vi "JKI_Test.vi"() -> ()   [LabVIEW 2018]
uses:
  Typedefs/DataBuffer.ctl
  <vilib>/xnet/xnet.llb/XNET Frame CAN.ctl
  <vilib>/xnet/xnet.llb/XNET Frame Type CAN.ctl
  TEST/Typedefs/Command.ctl
  <vilib>/xnet/xnet.llb/XNET Write (Frame CAN).vi
  <vilib>/xnet/xnet.llb/XNET Read (Frame CAN).vi
panel:
  out "Event":string
  out "CAN Data":string[][](table)
  out "Response Good?":bool
  in  "SendCan":bool
  in  "OK":bool
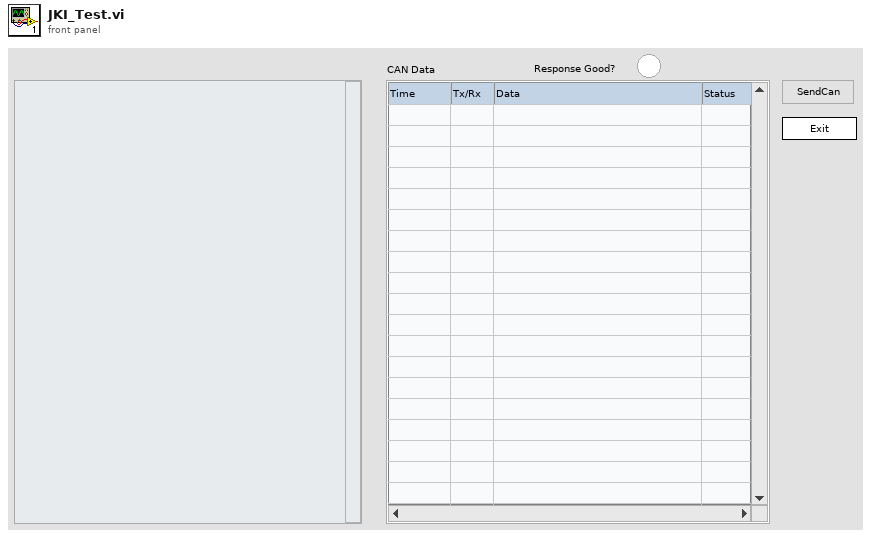
[diagram p1: front panel]
types:
  T1 = enum32{"Invalid", "Standard", "Closed", "Hidden", "Minimized", "Maximized"}
  T2 = enum32{"invalid app kind", "Development System", "Run Time System", "Student Edition", "Embedded LabVIEW", "Evaluation", "Custom"}
  T3 = typedef "DataBuffer.ctl" = cluster{"HMI":cluster{"Download Progress":refnum<vi>, "Status":refnum<vi>, "SCU Info":refnum<vi>, "PartType":refnum<vi>}, "path":path, "CAN":cluster{"Write Session in":refnum<k21>, "Read Session in":refnum<k21>, "TxRx Data":string[][], "Response Good?":bool, "spreadsheet string":string, "Rx Message":u8[], "CAN frame":T4, "HoldSession":refnum<k21>}, "error":errorcluster, "CaseControl":T6, "NewEvent":T8, "Byte Log":string[][], "Message":refnum<vi>}
  T4 = typedef "XNET Frame CAN.ctl" = cluster{"timestamp":timestamp, "payload":u8[], "identifier":u32, "type":T5, "extended?":bool, "echo?":bool}
  T5 = typedef "XNET Frame Type CAN.ctl" = u8
  T6 = typedef "CaseControl.ctl" = cluster{"histCase":cluster{"time":string, "event":T7, "pass?":bool}[], "retryCount":i32, "presentCase":T7, "nextEvent":T7}
  T7 = typedef "Command.ctl" = enum16{"Extend Session: 10 83", "Tester Present: 3E 80", "Resquest Seed: 27 01", "Send Key: 27 02", "Check FBL:  31 01 FD 02", "Control DTC: 85 82", "Comm Control: 28 83 01", "Program Session Request: 10 02", "Request Seed: 27 35", "Seed Key: 27 36", "Request Download: 34 00 44", "Transfer Data: 36 XX YY", "More Data?", "Request Transfer Exit: 37", "Check Flash Driver Validity: 01 FD 03", "More Segment?", "Write Data Fingereint: 23 F1 F0+26", "EraseFlashMemory Routine: 31 01 FD 00 44", "More segment?(each file)", "CheckAppSwAppData Validity: 31 01 FD 04 44", "CheckAppSwAppData Dependency: 31 01 fd 01", "ECU Reset: 11 81", "System: Init", "System: Idle", "System: Error", "System: Wait", "System: Delay", "System: CAN Send 1", "System: CAN Send 2", "System: CAN Read", "System: Exit"}
  T8 = typedef "NewEvent.ctl" = cluster{"Delay_ms":i32, "Case":T7, "Payload":u8[], "Identifier":u32}
  T9 = cluster{"Core":cluster{"Current VI Reference":refnum<vi>, "Close Panel on Exit?":bool}, "Your Boolean data":bool, "Event":string, "Hist Event":string, "DataBuffer":T3, "Delay_ms":u32}
  T10 = cluster{"Current VI Reference":refnum<vi>, "Close Panel on Exit?":bool}
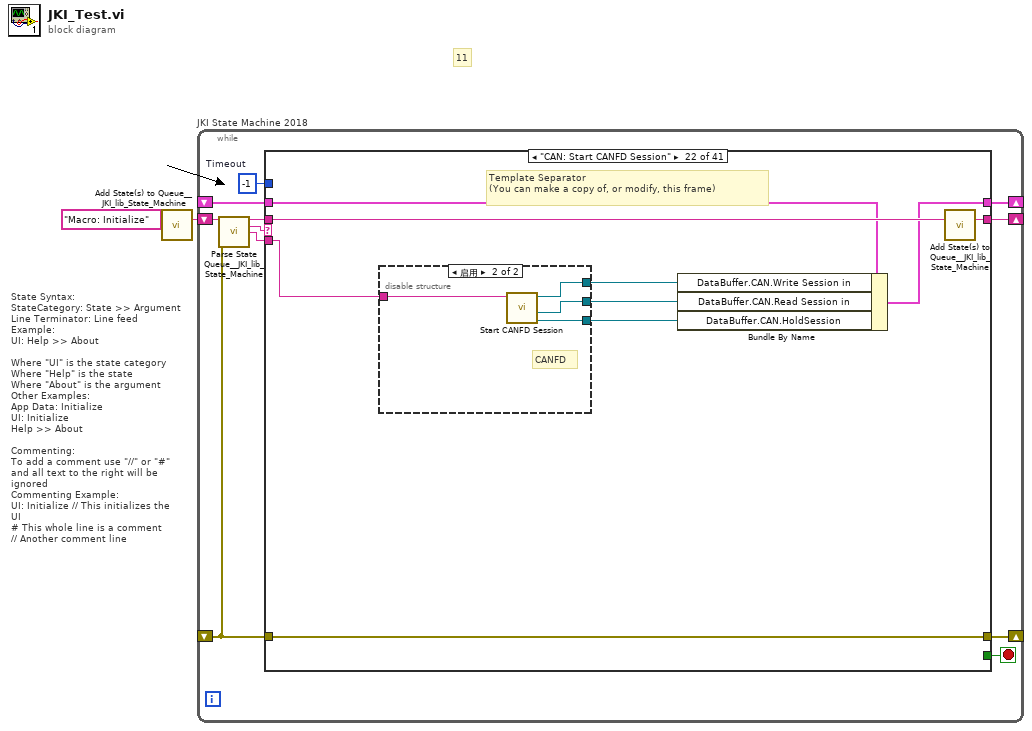
[diagram p0: block diagram]
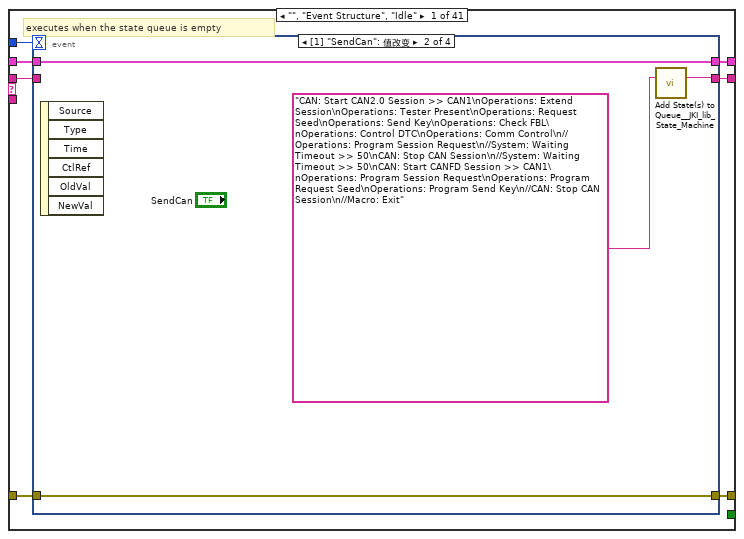
[diagram p2: hidden frame]
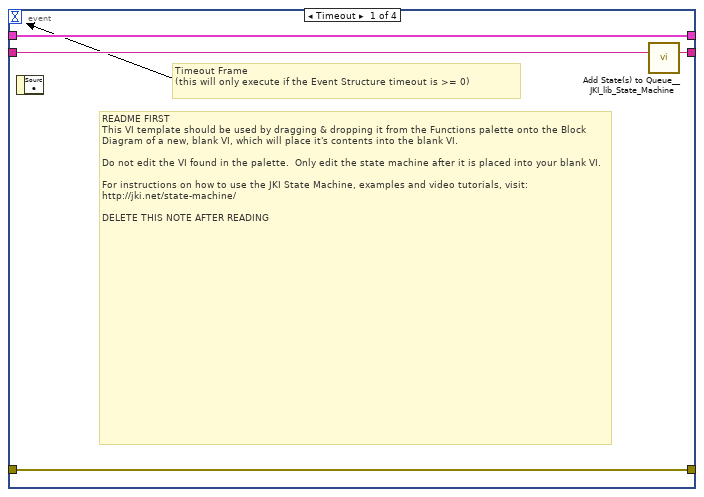
[diagram p3: hidden frame]
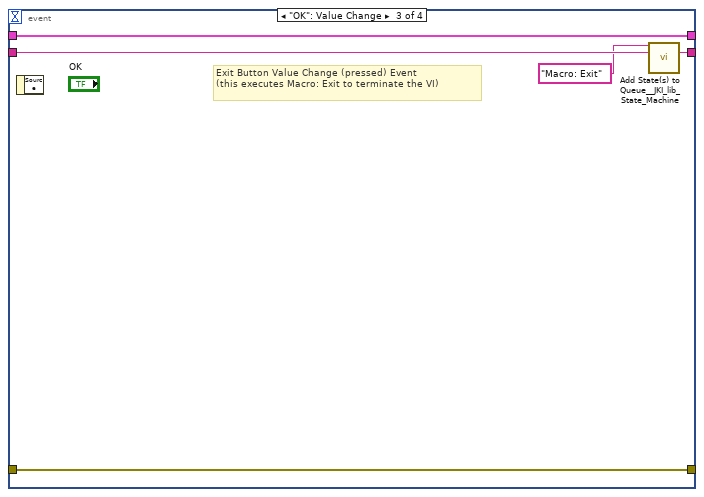
[diagram p4: hidden frame]
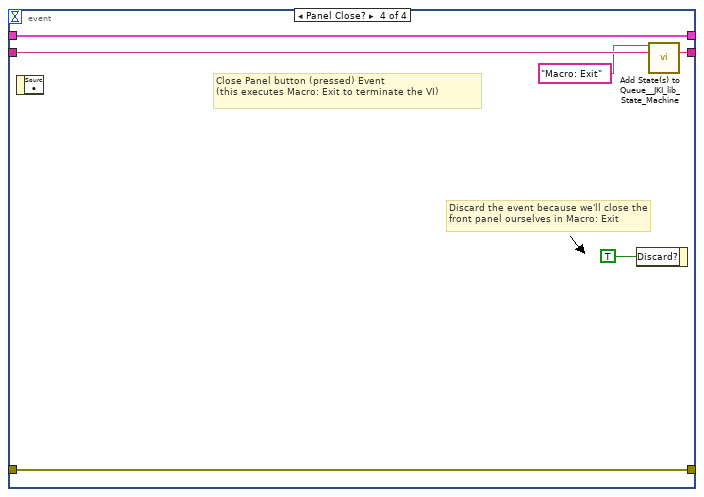
[diagram p5: hidden frame]
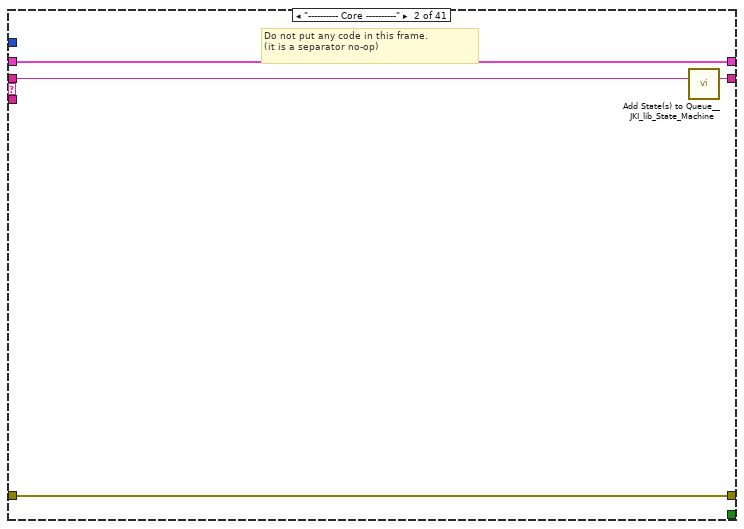
[diagram p6: hidden frame]
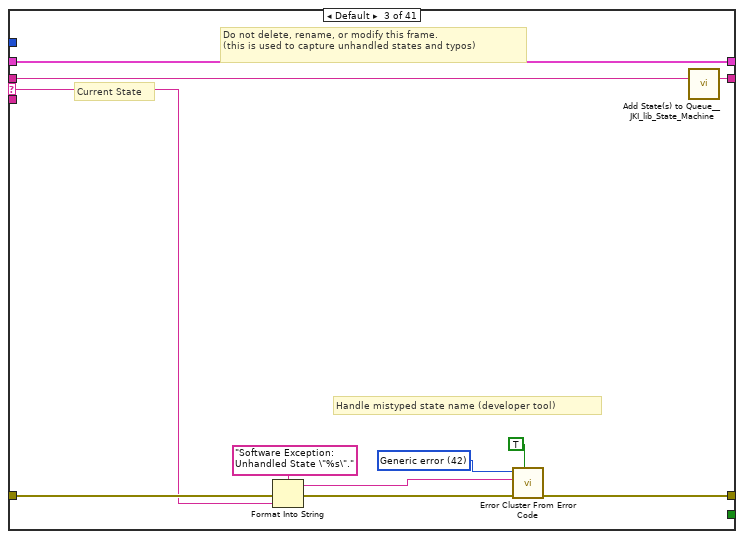
[diagram p7: hidden frame]
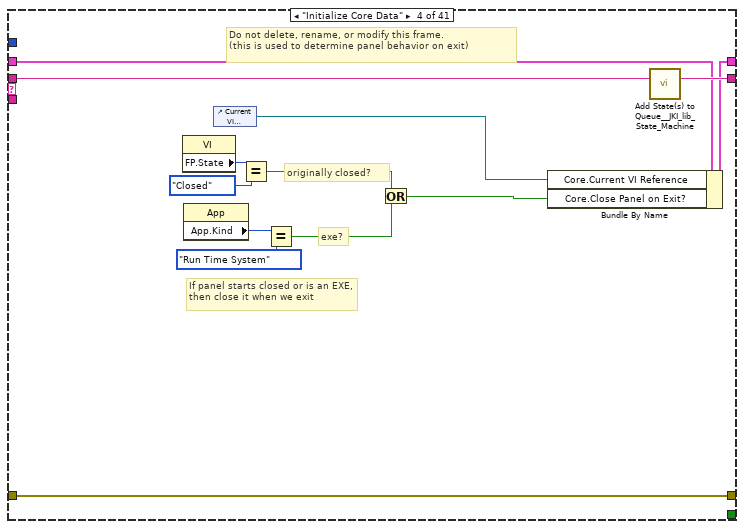
[diagram p8: hidden frame]
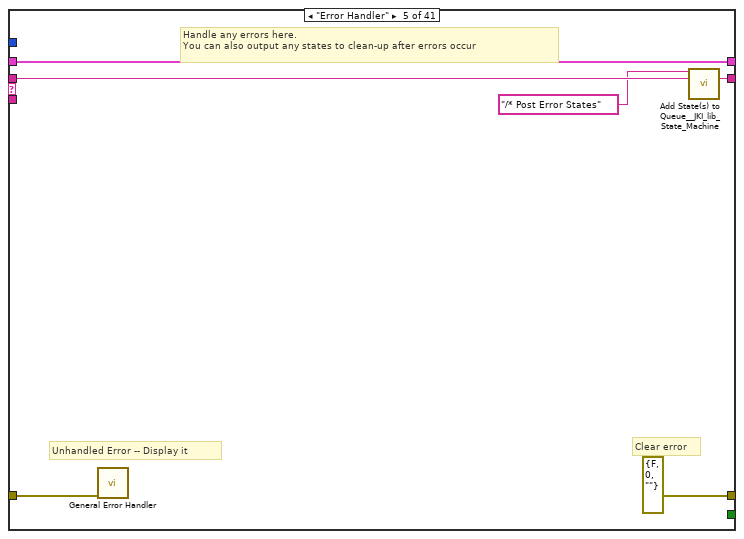
[diagram p9: hidden frame]
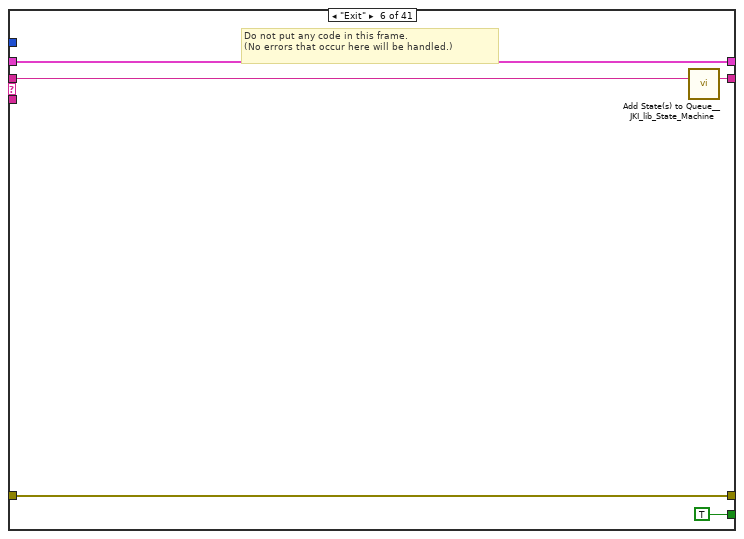
[diagram p10: hidden frame]
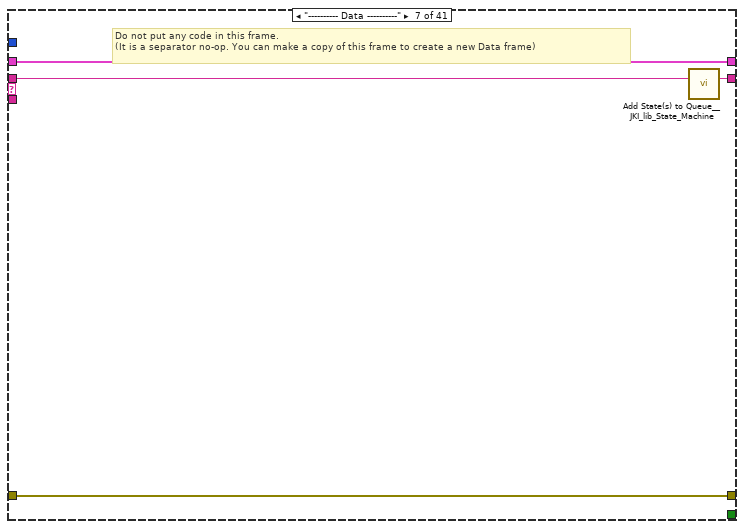
[diagram p11: hidden frame]
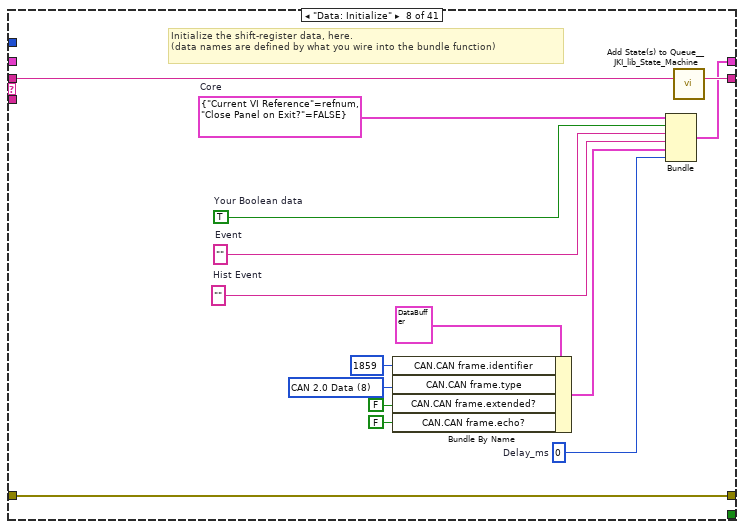
[diagram p12: hidden frame]
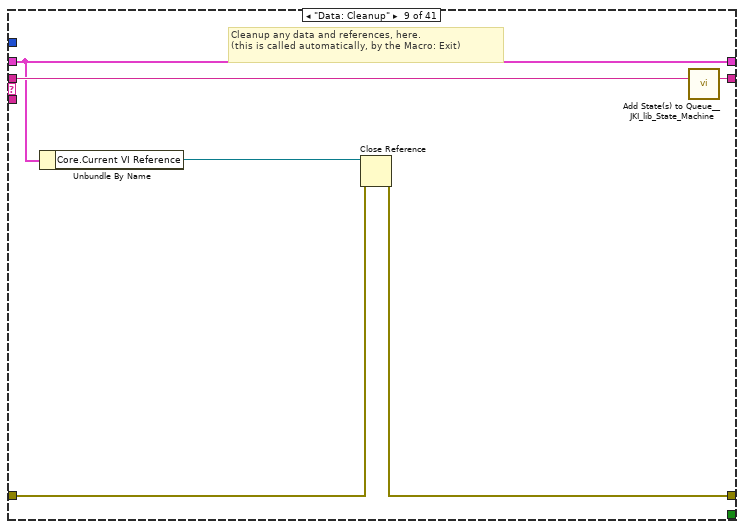
[diagram p13: hidden frame]
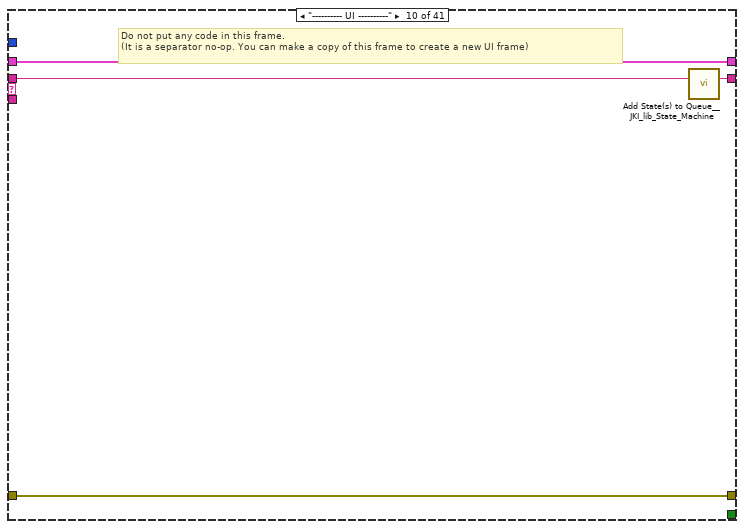
[diagram p14: hidden frame]
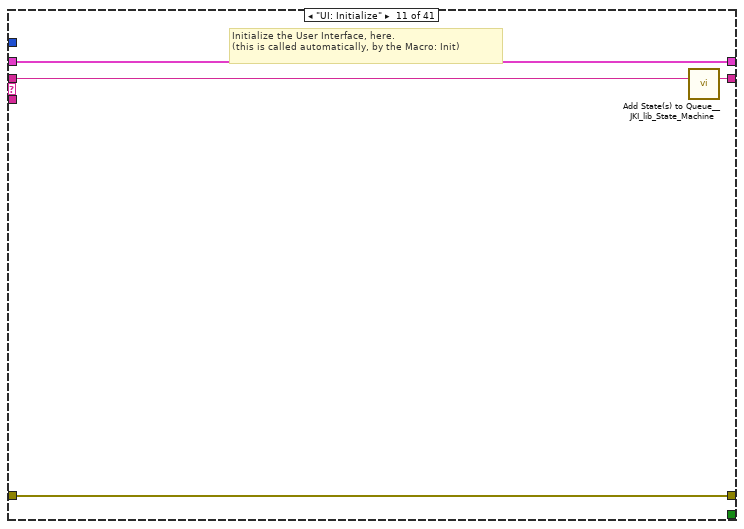
[diagram p15: hidden frame]
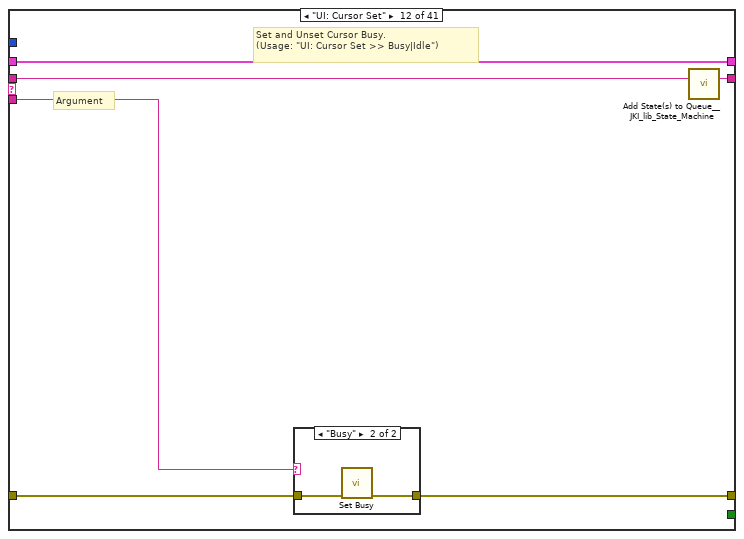
[diagram p16: hidden frame]
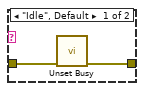
[diagram p17: hidden frame]
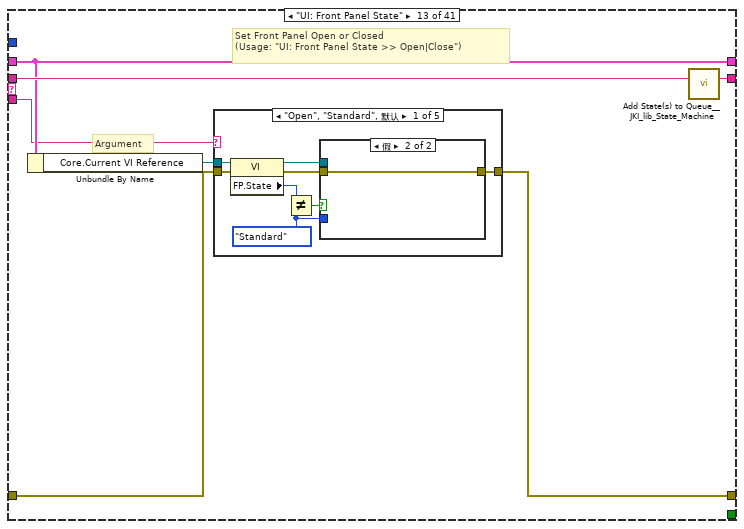
[diagram p18: hidden frame]
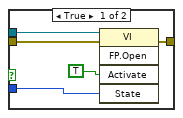
[diagram p19: hidden frame]
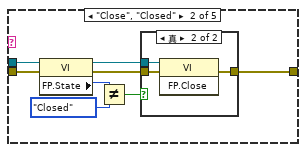
[diagram p20: hidden frame]
diagram:
  # "11"
  # "State Syntax:\nStateCategory: State >> Argument\nLine Terminator: Line feed\nExample:\nUI: Help >> About\n\nWhere \"UI\" is the state category\nWhere \"Help\" is the state\nWhere \"About\" is the argument\nOther Examples:\nApp Data: Initialize\nUI: Initialize\nHelp >> About\n\nCommenting:\nTo add a comment use \"//\" or \"#\" and all text to the right will be ignored\nCommenting Example:\nUI: Initialize // This initializes the UI\n# This whole line is a comment\n// Another comment line"
  n1 = call <vilib>:"Add State(s) to Queue__JKI_lib_State_Machine.vi"("State(s) in (\"\")"="Macro: Initialize") -> ("States Out"=w2:string)  [unwired: 14 in]
  n2 = while "JKI State Machine 2018" {
    shift-right: [w6] -> _
    shift-left: _ -> [w5]
    shift-right: [w9] -> _
    shift-left: _ -> [w3]
    shift-right: [w8] -> _
    shift-left: w2 -> [w10]
    stop <- w7 stop-if-true
    w4 = -1  # Timeout
    n3 = call <vilib>:"Parse State Queue__JKI_lib_State_Machine.vi"("State Queue"=w10, "Error In (no error)"=w3) -> ("Remaining States"=w12:string, "Current State"=w13:string, "Arguments"=w11:string)  [unwired: 11 in]
    n4 = case shown="\"CAN: Start CANFD Session\"" w13 {
      selector: w13 -> [_ _ w44 _ _ _ _ _ _ _ _ _ _ _ _ _ _ _ _ _ _ _ _ _ _ _ _ _ _ _ _ w363 w383 w404 w424 w448 w468 w491 w511 w532 w553]
      tunnel: w12 -> [w20 w43 w48 w67 w73 w78 w82 w97 w103 w107 w111 w117 w128 w197 w202 w212 w216 w236 w250 w254 w263 w279 w301 w319 w333 w339 w343 w347 w351 w355 w359 w380 w401 w421 w445 w465 w486 w506 w527 w549 w574]
      tunnel: w11 -> [_ _ _ _ _ _ _ _ _ _ _ w112 w122 _ _ _ _ _ w240 _ w257 w273 w295 _ _ _ _ _ _ _ _ w361 w382 w403 w423 w447 w467 w490 w510 w531 w552]
      tunnel: w5 -> [w18 w40 w46 w60 w70 w76 w79 _ w98 w104 w109 w115 w124 w194 w199 w209 w213 w233 w247 w251 w261 w277 w298 w316 w331 w336 w340 w344 w348 w352 w356 w372 w393 w413 w437 w457 w478 w498 w519 w541 w566]
      tunnel: [w17 w41 w50 w64 errorcluster {"status"=FALSE, "code"=0, "source"=""} ("error out") w75 w80 w94 w99 w105 w108 w113 w125 w195 w200 w210 w214 w234 w248 w252 w255 w271 w299 w317 w327 w337 w341 w345 w349 w353 w357 w378 w399 w419 w443 w463 w484 w504 w525 w547 w572] -> w9
      tunnel: w3 -> [w16 w41 w49 w64 w69 w75 w80 w94 w100 w105 w108 w114 w126 w195 w200 w210 w214 _ w248 w252 w255 w271 w299 w317 w327 w337 w341 w345 w349 w353 w357 w378 w399 w419 w443 w463 w484 w504 w525 w547 w572]
      tunnel: [w19 w42 w47 w66 w72 w77 w81 w96 w102 w106 w110 w116 w127 w196 w201 w211 w215 w235 w249 w253 w262 w278 w300 w318 w332 w338 w342 w346 w350 w354 w358 w379 w400 w420 w444 w464 w485 w505 w526 w548 w573] -> w8
      tunnel: [_ _ _ _ _ TRUE _ _ _ _ _ _ _ _ _ _ _ _ _ _ _ _ _ _ _ _ _ _ _ _ _ _ _ _ _ _ _ _ _ _ _] -> w7
      tunnel: [w15 w40 w46 w65 w70 w76 w79 w95 w98 w104 w109 w115 w124 w194 w199 w209 w213 w232 w247 w251 w260 w276 w297 w316 w331 w336 w340 w344 w348 w352 w356 w371 w392 w412 w436 w456 w477 w497 w518 w540 w565] -> w6
      tunnel: w4 -> [w14 _ _ _ _ _ _ _ _ _ _ _ _ _ _ _ _ _ _ _ _ _ _ _ _ _ _ _ _ _ _ _ _ _ _ _ _ _ _ _ _]
      frame "", "Event Structure", "Idle" {
        # "executes when the state queue is empty"
        n5 = event shown="[1] \"SendCan\": 值改变" {
          selector: _ -> [_ _ _ _]
          dyn-events: _ -> [_ _ _ _]
          timeout: w14 -> [_ _ _ _]
          tunnel: w20 -> [w24 _ w33 w39]
          tunnel: [w23 w27 w32 w38] -> w19
          tunnel: w18 -> [w21 w28 w30 w36]
          tunnel: [w22 w26 w31 w37] -> w17
          tunnel: w16 -> [w22 w26 w31 w37]
          tunnel: [w21 w28 w30 w36] -> w15
          event Timeout {
            # "README FIRST\nThis VI template should be used by dragging & dropping it from the Functions palette onto the Block Diagram of a new, blank VI, which will place it's contents into the blank VI.\n\nDo not edit the VI found in the palette.  Only edit the state machine after it is placed into your blank VI.\n\nFor instructions on how to use the JKI State Machine, examples and video tutorials, visit:\nhttp://jki.net/state-machine/\n\nDELETE THIS NOTE AFTER READING"
            # "Timeout Frame\n(this will only execute if the Event Structure timeout is >= 0)"
            n6 = event-data() -> ()  [unwired: 1 in, 1 out]
            n7 = call <vilib>:"Add State(s) to Queue__JKI_lib_State_Machine.vi"("State(s) in (\"\")"=w24) -> ("States Out"=w23:string)  [unwired: 14 in]
          }
          event "SendCan": Value Change {
            n8 = event-data() -> ()  [unwired: 1 in, 6 out]
            n9 = call <vilib>:"Add State(s) to Queue__JKI_lib_State_Machine.vi"("State(s) in (\"\")"="CAN: Start CAN2.0 Session >> CAN1\nOperations: Extend Session\nOperations: Tester Present\nOperations: Request Seed\nOperations: Send Key\nOperations: Check FBL\nOperations: Control DTC\nOperations: Comm Control\n//Operations: Program Session Request\n//System: Waiting Timeout >> 50\nCAN: Stop CAN Session\n//System: Waiting Timeout >> 50\nCAN: Start CANFD Session >> CAN1\nOperations: Program Session Request\nOperations: Program Request Seed\nOperations: Program Send Key\n//CAN: Stop CAN Session\n//Macro: Exit") -> ("States Out"=w27:string)  [unwired: 14 in]
          }
          event "OK": Value Change {
            # "Exit Button Value Change (pressed) Event\n(this executes Macro: Exit to terminate the VI)"
            n10 = event-data() -> ()  [unwired: 1 in, 1 out]
            n11 = call <vilib>:"Add State(s) to Queue__JKI_lib_State_Machine.vi"("State(s) in Front (\"\")"="Macro: Exit", "State(s) in (\"\")"=w33) -> ("States Out"=w32:string)  [unwired: 13 in]
          }
          event Panel Close? {
            # "Discard the event because we'll close the front panel ourselves in Macro: Exit"
            # "Close Panel button (pressed) Event\n(this executes Macro: Exit to terminate the VI)"
            n12 = event-data() -> ()  [unwired: 1 in, 1 out]
            n13 = event-data("Discard?"=TRUE) -> ()  [unwired: 1 in, 1 out]
            n14 = call <vilib>:"Add State(s) to Queue__JKI_lib_State_Machine.vi"("State(s) in Front (\"\")"="Macro: Exit", "State(s) in (\"\")"=w39) -> ("States Out"=w38:string)  [unwired: 13 in]
          }
        }
      }
      frame "---------- Core ----------" {
        # "Do not put any code in this frame.\n(it is a separator no-op)"
        n15 = call <vilib>:"Add State(s) to Queue__JKI_lib_State_Machine.vi"("State(s) in (\"\")"=w43) -> ("States Out"=w42:string)  [unwired: 14 in]
      }
      frame Default {
        w53 = 42 items=["No error", "Argument error", "Memory is full", "Out of zone", "End of file", "File already open", "Generic file I/O error", "File not found", "File permission error", "Disk is full", "Duplicate path", "Too many files open", "System feature not enabled", "Resource file not found", "Cannot add resource", "Resource not found", "Image not found", "Image memory error", "Pen does not exist", "Config type invalid", "Config token not found", "Config parse error", "Config memory error", "Bad external code format", "Bad external code offset", "External code not present", "Null window", "Destroy window error", "Null menu", "Print aborted", "Bad print record", "Print driver error", "Windows error during printing", "Memory error during printing", "Print dialog error", "Generic print error", "Invalid device refnum", "Device not found", "Device parameter error", "Device unit error", "Cannot open device", "Device call aborted", "Generic error", "Cancelled by user", "Object ID too low", "Object ID too high", "Object not in heap", "Unknown heap", "Unknown object (invalid DefProc)", "Unknown object (DefProc not in table)", "Message out of range", "Invalid (null) method", "Unknown message", "Manager call not supported", "Bad address", "Network operation in progress", "Network operation timed out", "Connection is busy", "Network attribute not supported", "Network error", "Address in use", "System out of memory", "Connection aborted", "Connection refused", "Not connected", "Already connected", "Connection closed", "Initialization error (interapplication manager)", "Bad occurrence", "Wait on unbound occurrence handler", "Occurrence queue overflow", "Datalog type conflict", "Unused", "Unrecognized type (interapplication manager)", "Memory corrupt", "Failed to make temporary DLL", "Old CIN version", "Drag socket not found", "Failed to load drop-object", "Failed to register OLE object", "Failed to release OLE object", "Format specifier type mismatch", "Unknown format specifier", "Too few format specifiers", "Too many format specifiers", "Scan failed", "Newer CIN version", "Error converting to variant", "Runtime menu error", "Password tampered", "Variant attribute not found", "Incompatible variant data type", "Event data is not available", "Event Store is not present", "Occurrence is not found", "Event Queue is not created", "Event info is not available", "Refnum passed is NULL", "Error retrieving Class GUID", "Error retrieving CoClass GUID", "Error retrieving TypeLib GUID.", "Bad built application magic bytes.", "Specific driver is different from the specific driver associated with the Logical Name.", "There is no session opened to the class driver.", "Max Error", "MAX - Error with config objects", "MAX - Error loading configuration", "MAX - Group not supported"]
        # "Current State"
        # "Do not delete, rename, or modify this frame.\n(this is used to capture unhandled states and typos)"
        # "Handle mistyped state name (developer tool)"
        n16 = Format Into String(format string="Software Exception: Unhandled State \"%s\"." ("message"), error in=w49, w44) -> (resulting string=w52:string, error out=w51:errorcluster)  [unwired: 1 in]
        n17 = call <vilib>:"Error Cluster From Error Code.vi"("show call chain? (False)"=TRUE, "error in (no error)"=w51, "error message (\"\")"=w52, "error code (0)"=w53) -> ("error out"=w50:errorcluster)  [unwired: 5 in]
        n18 = call <vilib>:"Add State(s) to Queue__JKI_lib_State_Machine.vi"("State(s) in (\"\")"=w48) -> ("States Out"=w47:string)  [unwired: 14 in]
      }
      frame "Initialize Core Data" {
        # "Do not delete, rename, or modify this frame.\n(this is used to determine panel behavior on exit)"
        # "originally closed?"
        # "exe?"
        # "If panel starts closed or is an EXE, then close it when we exit"
        n19 = property class="VI"() -> ("FP.State"=w57:T1)  [unwired: 2 in, 2 out]
        n20 = property class="App"() -> ("App.Kind"=w63:T2)  [unwired: 2 in, 2 out]
        n21 = control-ref of="Current VI Reference"() -> (w58:refnum<vi>)
        n22 = Equal?(x=w57, y=T1."Closed" ("Front Panel Window:State")) -> (x = y?=w55:bool)
        n23 = Equal?(x=w63, y=T2."Run Time System" ("Application:Kind")) -> (x = y?=w61:bool)
        n24 = Or(x=w55, y=w61) -> (x .or. y?=w59:bool)
        n25 = Bundle By Name(cluster=w60, "Core.Current VI Reference"=w58, "Core.Close Panel on Exit?"=w59) -> (w65:T9)
        n26 = call <vilib>:"Add State(s) to Queue__JKI_lib_State_Machine.vi"("State(s) in (\"\")"=w67) -> ("States Out"=w66:string)  [unwired: 14 in]
      }
      frame "Error Handler" {
        # "Unhandled Error -- Display it"
        # "Handle any errors here.\nYou can also output any states to clean-up after errors occur"
        # "Clear error"
        n27 = call <vilib>:"General Error Handler.vi"("error in (no error)"=w69) -> ()  [unwired: 10 in, 5 out]
        n28 = call <vilib>:"Add State(s) to Queue__JKI_lib_State_Machine.vi"("State(s) in Front (\"\")"="/* Post Error States", "State(s) in (\"\")"=w73) -> ("States Out"=w72:string)  [unwired: 13 in]
      }
      frame "Exit" {
        # "Do not put any code in this frame.\n(No errors that occur here will be handled.)"
        n29 = call <vilib>:"Add State(s) to Queue__JKI_lib_State_Machine.vi"("State(s) in (\"\")"=w78) -> ("States Out"=w77:string)  [unwired: 14 in]
      }
      frame "---------- Data ----------" {
        # "Do not put any code in this frame.\n(It is a separator no-op. You can make a copy of this frame to create a new Data frame)"
        n30 = call <vilib>:"Add State(s) to Queue__JKI_lib_State_Machine.vi"("State(s) in (\"\")"=w82) -> ("States Out"=w81:string)  [unwired: 14 in]
      }
      frame "Data: Initialize" {
        w83 = u32 0  # Delay_ms
        w84 = ""  # Hist Event
        w87 = T5 8 items=["CAN Data"=0, "CAN Remote"=1, "CAN Bus Error"=2, "CAN 2.0 Data"=8, "CAN FD Data"=16, "CAN FD+BRS Data"=24, "J1939 Data"=192, "Delay"=224, "Log Trigger"=225, "Start Trigger"=226] ("CAN.CAN frame.type")
        w91 = T10 {"Current VI Reference"=refnum, "Close Panel on Exit?"=FALSE}  # Core
        w93 = TRUE  # Your Boolean data
        w92 = ""  # Event
        # "Initialize the shift-register data, here.\n(data names are defined by what you wire into the bundle function)"
        n31 = Bundle By Name(cluster=T3 {"HMI"={"Download Progress"=refnum, "Status"=refnum, "SCU Info"=refnum, "PartType"=refnum}, "path"=path "", "CAN"={"Write Session in"="", "Read Session in"="", "TxRx Data"=[], "Response Good?"=FALSE, "spreadsheet string"="", "Rx Message"=[], "CAN frame"={"timestamp"=timestamp(0 s since 1904-01-01), "payload"=[2, 39, 3, 85, 85, 85, 85, 85], "identifier"=402391172, "type"=16, "extended?"=TRUE, "echo?"=FALSE}, "HoldSession"=""}, "error"={"status"=FALSE, "code"=0, "source"=""}, "CaseControl"={"histCase"=[], "retryCount"=0, "presentCase"=enum."Extend Session: 10 83", "nextEvent"=enum."Extend Session: 10 83"}, "NewEvent"={"Delay_ms"=0, "Case"=enum."Extend Session: 10 83", "Payload"=[], "Identifier"=0}, "Byte Log"=[], "Message"=refnum} ("DataBuffer"), "CAN.CAN frame.identifier"=u32 1859, "CAN.CAN frame.type"=w87, "CAN.CAN frame.extended?"=FALSE, "CAN.CAN frame.echo?"=FALSE) -> (w89:T3)
        n32 = Bundle("Core"=w91, "Your Boolean data"=w93, "Event"=w92, "Hist Event"=w84, "DataBuffer"=w89, "Delay_ms"=w83) -> (w95:T9)  [unwired: 1 in]
        n33 = call <vilib>:"Add State(s) to Queue__JKI_lib_State_Machine.vi"("State(s) in (\"\")"=w97) -> ("States Out"=w96:string)  [unwired: 14 in]
      }
      frame "Data: Cleanup" {
        # "Cleanup any data and references, here.\n(this is called automatically, by the Macro: Exit)"
        n34 = Unbundle By Name(w98) -> ("Core.Current VI Reference"=w101:refnum<vi>)
        n35 = Close Reference(reference=w101, error in (no error)=w100) -> (error out=w99:errorcluster)
        n36 = call <vilib>:"Add State(s) to Queue__JKI_lib_State_Machine.vi"("State(s) in (\"\")"=w103) -> ("States Out"=w102:string)  [unwired: 14 in]
      }
      frame "---------- UI ----------" {
        # "Do not put any code in this frame.\n(It is a separator no-op. You can make a copy of this frame to create a new UI frame)"
        n37 = call <vilib>:"Add State(s) to Queue__JKI_lib_State_Machine.vi"("State(s) in (\"\")"=w107) -> ("States Out"=w106:string)  [unwired: 14 in]
      }
      frame "UI: Initialize" {
        # "Initialize the User Interface, here.\n(this is called automatically, by the Macro: Init)"
        n38 = call <vilib>:"Add State(s) to Queue__JKI_lib_State_Machine.vi"("State(s) in (\"\")"=w111) -> ("States Out"=w110:string)  [unwired: 14 in]
      }
      frame "UI: Cursor Set" {
        # "Argument"
        # "Set and Unset Cursor Busy.\n(Usage: \"UI: Cursor Set >> Busy|Idle\")"
        n39 = case shown="\"Busy\"" w112 {
          tunnel: w114 -> [w119 w121]
          tunnel: [w118 w120] -> w113
          frame "Idle", Default {
            n40 = call <vilib>:"Unset Busy.vi"("error in (no error)"=w119) -> ("error out"=w118:errorcluster)  [unwired: 10 in]
          }
          frame "Busy" {
            n41 = call <vilib>:"Set Busy.vi"("error in (no error)"=w121) -> ("error out"=w120:errorcluster)  [unwired: 9 in, 1 out]
          }
        }
        n42 = call <vilib>:"Add State(s) to Queue__JKI_lib_State_Machine.vi"("State(s) in (\"\")"=w117) -> ("States Out"=w116:string)  [unwired: 14 in]
      }
      frame "UI: Front Panel State" {
        # "Argument"
        # "Set Front Panel Open or Closed\n(Usage: \"UI: Front Panel State >> Open|Close\")"
        n43 = Unbundle By Name(w124) -> ("Core.Current VI Reference"=w123:refnum<vi>)
        n44 = case shown="\"Open\", \"Standard\", 默认" w122 {
          tunnel: w126 -> [w134 w149 w160 w173 w186]
          tunnel: [w136 w150 w162 w175 w188] -> w125
          tunnel: w123 -> [w135 w147 w161 w174 w187]
          frame "Open", "Standard", Default {
            w129 = T1."Standard" ("State")
            n45 = property class="VI"(reference=w135, error in=w134) -> (reference out=w132:refnum<vi>, error out=w133:errorcluster, "FP.State"=w131:T1)
            n46 = Not Equal?(x=w131, y=w129) -> (x != y?=w130:bool)
            n47 = case shown="假" w130 {
              tunnel: [w140 w142] -> w136
              tunnel: w133 -> [w139 w142]
              tunnel: w132 -> [w138 _]
              tunnel: w129 -> [w137 _]
              frame True {
                n48 = invoke class="VI" method="FP.Open"(reference=w138, error in=w139, "Activate"=TRUE, "State"=w137) -> (error out=w140:errorcluster)  [unwired: 1 in, 4 out]
              }
              frame False {
              }
            }
          }
          frame "Close", "Closed" {
            n49 = property class="VI"(reference=w147, error in=w149) -> (reference out=w146:refnum<vi>, error out=w148:errorcluster, "FP.State"=w144:T1)
            n50 = Not Equal?(x=w144, y=T1."Closed" ("Front Panel Window:State")) -> (x != y?=w143:bool)
            n51 = case shown="真" w143 {
              tunnel: [w151 w154] -> w150
              tunnel: w148 -> [w151 w153]
              tunnel: w146 -> [_ w152]
              frame False {
              }
              frame True {
                n52 = invoke class="VI" method="FP.Close"(reference=w152, error in=w153) -> (error out=w154:errorcluster)  [unwired: 1 in, 2 out]
              }
            }
          }
          frame "Hidden", "Hide" {
            w155 = T1."Hidden" ("State")
            n53 = property class="VI"(reference=w161, error in=w160) -> (reference out=w158:refnum<vi>, error out=w159:errorcluster, "FP.State"=w157:T1)
            n54 = Not Equal?(x=w157, y=w155) -> (x != y?=w156:bool)
            n55 = case shown="假" w156 {
              tunnel: [w166 w167] -> w162
              tunnel: w159 -> [w165 w167]
              tunnel: w158 -> [w164 _]
              tunnel: w155 -> [w163 _]
              frame True {
                n56 = invoke class="VI" method="FP.Open"(reference=w164, error in=w165, "State"=w163) -> (error out=w166:errorcluster)  [unwired: 2 in, 4 out]
              }
              frame False {
              }
            }
          }
          frame "Minimize", "Minimized" {
            w168 = T1."Minimized" ("State")
            n57 = property class="VI"(reference=w174, error in=w173) -> (reference out=w171:refnum<vi>, error out=w172:errorcluster, "FP.State"=w170:T1)
            n58 = Not Equal?(x=w170, y=w168) -> (x != y?=w169:bool)
            n59 = case shown="真" w169 {
              tunnel: [w179 w180] -> w175
              tunnel: w172 -> [w178 w180]
              tunnel: w171 -> [w177 _]
              tunnel: w168 -> [w176 _]
              frame True {
                n60 = invoke class="VI" method="FP.Open"(reference=w177, error in=w178, "State"=w176) -> (error out=w179:errorcluster)  [unwired: 2 in, 4 out]
              }
              frame False {
              }
            }
          }
          frame "Maximize", "Maximized" {
            w181 = T1."Maximized" ("State")
            n61 = property class="VI"(reference=w187, error in=w186) -> (reference out=w184:refnum<vi>, error out=w185:errorcluster, "FP.State"=w183:T1)
            n62 = Not Equal?(x=w183, y=w181) -> (x != y?=w182:bool)
            n63 = case shown="真" w182 {
              tunnel: [w192 w193] -> w188
              tunnel: w185 -> [w191 w193]
              tunnel: w184 -> [w190 _]
              tunnel: w181 -> [w189 _]
              frame True {
                n64 = invoke class="VI" method="FP.Open"(reference=w190, error in=w191, "State"=w189) -> (error out=w192:errorcluster)  [unwired: 2 in, 4 out]
              }
              frame False {
              }
            }
          }
        }
        n65 = call <vilib>:"Add State(s) to Queue__JKI_lib_State_Machine.vi"("State(s) in (\"\")"=w128) -> ("States Out"=w127:string)  [unwired: 14 in]
      }
      frame "---------- Macro ----------" {
        # "Do not put any code in this frame.\n(It is a separator no-op. You can make a copy of this frame to create a new Macro frame)"
        n66 = call <vilib>:"Add State(s) to Queue__JKI_lib_State_Machine.vi"("State(s) in (\"\")"=w197) -> ("States Out"=w196:string)  [unwired: 14 in]
      }
      frame "Macro: Initialize" {
        # "Initialization Macro\n(This is called once, when the VI starts)"
        n67 = call <vilib>:"Add State(s) to Queue__JKI_lib_State_Machine.vi"("State(s) in Front (\"\")"="Data: Initialize\nInitialize Core Data\nUI: Initialize\nUI: Front Panel State >> Open", "State(s) in (\"\")"=w202) -> ("States Out"=w201:string)  [unwired: 13 in]
      }
      frame "Macro: Exit" {
        # "Exit Macro\n(This is called once, when the VI exits)"
        n68 = Unbundle By Name(w209) -> ("Core.Close Panel on Exit?"=w208:bool)
        n69 = Select(t="UI: Front Panel State >> Close", s=w208, f="") -> (s? t:f=w205:string)
        n70 = call <vilib>:"Add State(s) to Queue__JKI_lib_State_Machine.vi"("State(s) in (\"\")"=w205, "State(s) at Back (\"\")"="Data: Cleanup\nExit") -> ("States Out"=w203:string)  [unwired: 13 in]
        n71 = call <vilib>:"Add State(s) to Queue__JKI_lib_State_Machine.vi"("State(s) in Front (\"\")"=w203, "State(s) in (\"\")"=w212) -> ("States Out"=w211:string)  [unwired: 13 in]
      }
      frame "---------- System ----------" {
        # "Do not put any code in this frame.\n(It is a separator no-op. You can make a copy of this frame to create a new Macro frame)"
        n72 = call <vilib>:"Add State(s) to Queue__JKI_lib_State_Machine.vi"("State(s) in (\"\")"=w216) -> ("States Out"=w215:string)  [unwired: 14 in]
      }
      frame "System: Updata Display" {
        # "Your code here.\n(You can make a copy of, or modify, this frame)"
        n73 = Unbundle By Name(w233) -> ("Hist Event"=w231:string, "Event"=w230:string, "DataBuffer.Byte Log"=w225:string[][], "DataBuffer.CAN.TxRx Data"=w223:string[][], "DataBuffer.CAN.Response Good?"=w227:bool, "DataBuffer.error"=w234:errorcluster)
        "Response Good?" <- w227
        n74 = Index Array(array=w223) -> (element=w222:string[])  [unwired: 2 in]
        n75 = Format Into String(w227) -> (resulting string=w218:string)  [unwired: 3 in, 1 out]
        n76 = Insert Into Array(array=w222, index=3 ("索引"), new element=w218) -> (w220:string[])
        n77 = Build Array(w220) -> (w219:string[][])
        n78 = Concatenate Strings(w231, w230, " -- | " ("字符串"), w218, "\r") -> (w228:string)
        "Event" <- w228
        n79 = Build Array (concatenate)(w225, w219) -> (w224:string[][])
        "CAN Data" <- w224
        n80 = Tick Count (ms)() -> (millisecond timer value=w217:u32)
        n81 = Bundle By Name(cluster=w233, "Hist Event"=w228, "DataBuffer.Byte Log"=w224, "Delay_ms"=w217) -> (w232:T9)
        n82 = call <vilib>:"Add State(s) to Queue__JKI_lib_State_Machine.vi"("State(s) in (\"\")"=w236) -> ("States Out"=w235:string)  [unwired: 14 in]
      }
      frame "System: Waiting Timeout" {
        # "Template Separator\n(You can make a copy of, or modify, this frame)"
        n83 = Decimal String To Number(string=w240) -> (number=w245:i32)  [unwired: 2 in, 1 out]
        n84 = Unbundle By Name(w247) -> ("Delay_ms"=w237:u32)
        n85 = Tick Count (ms)() -> (millisecond timer value=w238:u32)
        n86 = Subtract(x=w238, y=w237) -> (x-y=w246:u32)
        n87 = Greater Or Equal?(x=w246, y=w245) -> (x >= y?=w244:bool)
        n88 = Concatenate Strings("System: Waiting Timeout >> ", w240) -> (w239:string)
        n89 = Select(t="", s=w244, f=w239) -> (s? t:f=w243:string)
        n90 = call <vilib>:"Add State(s) to Queue__JKI_lib_State_Machine.vi"("State(s) in Front (\"\")"=w243, "State(s) in (\"\")"=w250) -> ("States Out"=w249:string)  [unwired: 13 in]
      }
      frame "---------- CAN ----------" {
        # "Template Separator\n(You can make a copy of, or modify, this frame)"
        n91 = call <vilib>:"Add State(s) to Queue__JKI_lib_State_Machine.vi"("State(s) in (\"\")"=w254) -> ("States Out"=w253:string)  [unwired: 14 in]
      }
      frame "CAN: Start CAN2.0 Session" {
        # "Template Separator\n(You can make a copy of, or modify, this frame)"
        n92 = disable-structure shown="启用" {
          disable-tunnel: [w266 w269] -> w259
          disable-tunnel: [w265 w268] -> w258
          disable-tunnel: w257 -> [w264 w270]
          disable-tunnel: [_ w267] -> w256
          frame Disabled {
            n93 = call "CAN Session.vi"("interface"=w264) -> ("read session"=w265:refnum<k21>, "write session"=w266:refnum<k21>)  [unwired: 8 in, 1 out]
          }
          frame Enabled {
            # "CAN2.0"
            n94 = call "Start CAN2.0 Session.vi"("CAN Interface"=w270) -> ("Tester Write Session out"=w267:refnum<k21>, "Read Session out"=w268:refnum<k21>, "DSC Write Session out"=w269:refnum<k21>)  [unwired: 8 in]
          }
        }
        n95 = Bundle By Name(cluster=w261, "DataBuffer.CAN.Write Session in"=w259, "DataBuffer.CAN.Read Session in"=w258, "DataBuffer.CAN.HoldSession"=w256) -> (w260:T9)
        n96 = call <vilib>:"Add State(s) to Queue__JKI_lib_State_Machine.vi"("State(s) in (\"\")"=w263) -> ("States Out"=w262:string)  [unwired: 14 in]
      }
      frame "CAN: Start CANFD Session" {
        # "Template Separator\n(You can make a copy of, or modify, this frame)"
        n97 = disable-structure shown="启用" {
          disable-tunnel: [w282 w286] -> w275
          disable-tunnel: [w281 w285] -> w274
          disable-tunnel: w273 -> [w280 w284]
          disable-tunnel: [_ w283] -> w272
          frame Disabled {
            n98 = call "CAN Session.vi"("interface"=w280) -> ("read session"=w281:refnum<k21>, "write session"=w282:refnum<k21>)  [unwired: 8 in, 1 out]
          }
          frame Enabled {
            # "CANFD"
            n99 = call "Start CANFD Session.vi"("CAN Interface"=w284) -> ("Tester Write Session out"=w283:refnum<k21>, "Read Session out"=w285:refnum<k21>, "DSC Write Session out"=w286:refnum<k21>)  [unwired: 8 in]
          }
        }
        n100 = Bundle By Name(cluster=w277, "DataBuffer.CAN.Write Session in"=w275, "DataBuffer.CAN.Read Session in"=w274, "DataBuffer.CAN.HoldSession"=w272) -> (w276:T9)
        n101 = call <vilib>:"Add State(s) to Queue__JKI_lib_State_Machine.vi"("State(s) in (\"\")"=w279) -> ("States Out"=w278:string)  [unwired: 14 in]
      }
      frame "CAN: Send Message" {
        w287 = T5 8 items=["CAN Data"=0, "CAN Remote"=1, "CAN Bus Error"=2, "CAN 2.0 Data"=8, "CAN FD Data"=16, "CAN FD+BRS Data"=24, "J1939 Data"=192, "Delay"=224, "Log Trigger"=225, "Start Trigger"=226] ("type")
        # "Your code here.\n(You can make a copy of, or modify, this frame)"
        n102 = for {
          N: 8 -> [_]
          shift-right: [w307] -> _
          shift-left: w295 -> [w309]
          tunnel: [w302] -> w292 mode=indexing
          n103 = Match Pattern(string=w309, regular expression=" " ("正则表达式")) -> (before substring=w306:string, after substring=w307:string)  [unwired: 1 in, 2 out]
          n104 = Empty String/Path?(string/path=w306) -> (empty?=w305:bool)
          n105 = Hexadecimal String To Number(string=w306) -> (number=w304:u32)  [unwired: 2 in, 1 out]
          n106 = Select(t=u32 255, s=w305, f=w304) -> (s? t:f=w302:u32)
        }
        n107 = Unbundle By Name(w298) -> ("DataBuffer.CAN.Write Session in"=w294:refnum<k21>)
        n108 = Bundle By Name(cluster=T4 {"timestamp"=timestamp(0 s since 1904-01-01), "payload"=[], "identifier"=0, "type"=0, "extended?"=FALSE, "echo?"=FALSE} ("CAN frame"), "identifier"=u32 1859, "payload"=w292, "type"=w287) -> (w290:T4)
        n109 = Build Array(w290) -> (w289:T4[])
        n110 = call-poly <vilib>:"XNET Write.vi"("session in"=w294, "data"=w289) -> ("session out"=w288:refnum<k21>)  [unwired: 12 in, 1 out]
        n111 = Bundle By Name(cluster=w298, "DataBuffer.CAN.Write Session in"=w288) -> (w297:T9)
        n112 = call <vilib>:"Add State(s) to Queue__JKI_lib_State_Machine.vi"("State(s) in (\"\")"=w301) -> ("States Out"=w300:string)  [unwired: 14 in]
      }
      frame "CAN: Recive Message" {
        # "Your code here.\n(You can make a copy of, or modify, this frame)"
        n113 = Unbundle By Name(w316) -> ("DataBuffer.CAN.Read Session in"=w314:refnum<k21>)
        n114 = call-poly <vilib>:"XNET Read.vi"("session in"=w314) -> ("data"=w315:T4[])  [unwired: 11 in, 3 out]
        n115 = for {
          tunnel: w315 -> [w325] mode=indexing
          tunnel: [w325] -> _ mode=indexing if=w320
          tunnel: [w320] -> w313
          stop <- w320 stop-if-true
          n116 = Unbundle By Name(w325) -> ("payload"=w324:u8[])
          n117 = Index Array(array=w324, index=1 ("索引")) -> (element=w322:u8)
          n118 = Equal?(x=w322, y=u8 80) -> (x = y?=w320:bool)
        }
        n119 = Select(t="", s=w313, f="CAN: Recive Message" ("State(s) in Front (\"\")")) -> (s? t:f=w311:string)
        n120 = call <vilib>:"Add State(s) to Queue__JKI_lib_State_Machine.vi"("State(s) in Front (\"\")"=w311, "State(s) in (\"\")"=w319) -> ("States Out"=w318:string)  [unwired: 13 in]
      }
      frame "CAN: Stop CAN Session" {
        # "Template Separator\n(You can make a copy of, or modify, this frame)"
        n121 = Unbundle By Name(w331) -> ("DataBuffer.CAN.Write Session in"=w330:refnum<k21>, "DataBuffer.CAN.Read Session in"=w329:refnum<k21>, "DataBuffer.CAN.HoldSession"=w326:refnum<k21>)
        n122 = Build Array(w330, w329, w326) -> (w328:refnum<k21>[])
        n123 = for {
          tunnel: w328 -> [w335] mode=indexing
          n124 = call <vilib>:"XNET Stop.vi"("session in"=w335) -> ("session out"=w334:refnum<k21>)  [unwired: 13 in, 1 out]
          n125 = call <vilib>:"XNET Clear.vi"("session in"=w334) -> ()  [unwired: 14 in, 1 out]
        }
        n126 = call <vilib>:"Add State(s) to Queue__JKI_lib_State_Machine.vi"("State(s) in (\"\")"=w333) -> ("States Out"=w332:string)  [unwired: 14 in]
      }
      frame "---------- S7 ----------" {
        # "Template Separator\n(You can make a copy of, or modify, this frame)"
        n127 = call <vilib>:"Add State(s) to Queue__JKI_lib_State_Machine.vi"("State(s) in (\"\")"=w339) -> ("States Out"=w338:string)  [unwired: 14 in]
      }
      frame "S7: Start Connect" {
        # "Template Separator\n(You can make a copy of, or modify, this frame)"
        n128 = call <vilib>:"Add State(s) to Queue__JKI_lib_State_Machine.vi"("State(s) in (\"\")"=w343) -> ("States Out"=w342:string)  [unwired: 14 in]
      }
      frame "S7: Write Bool" {
        # "Template Separator\n(You can make a copy of, or modify, this frame)"
        n129 = call <vilib>:"Add State(s) to Queue__JKI_lib_State_Machine.vi"("State(s) in (\"\")"=w347) -> ("States Out"=w346:string)  [unwired: 14 in]
      }
      frame "S7: Read Bool" {
        # "Template Separator\n(You can make a copy of, or modify, this frame)"
        n130 = call <vilib>:"Add State(s) to Queue__JKI_lib_State_Machine.vi"("State(s) in (\"\")"=w351) -> ("States Out"=w350:string)  [unwired: 14 in]
      }
      frame "S7: Close Connect" {
        # "Template Separator\n(You can make a copy of, or modify, this frame)"
        n131 = call <vilib>:"Add State(s) to Queue__JKI_lib_State_Machine.vi"("State(s) in (\"\")"=w355) -> ("States Out"=w354:string)  [unwired: 14 in]
      }
      frame "---------- Operations ----------" {
        # "Template Separator\n(You can make a copy of, or modify, this frame)"
        n132 = call <vilib>:"Add State(s) to Queue__JKI_lib_State_Machine.vi"("State(s) in (\"\")"=w359) -> ("States Out"=w358:string)  [unwired: 14 in]
      }
      frame "Operations: Extend Session" {
        # "Your code here.\n(You can make a copy of, or modify, this frame)"
        n133 = Concatenate Strings(w363, " >> " ("字符串"), w361) -> (w360:string)
        n134 = Unbundle By Name(w372) -> ("DataBuffer.CAN.Write Session in"=w377:refnum<k21>, "DataBuffer.CAN.Read Session in"=w376:refnum<k21>, "DataBuffer.CAN.CAN frame"=w375:T4)
        n135 = Bundle By Name(cluster=w375, "payload"=u8[] [2, 16, 131, 170, 170, 170, 170, 170], "identifier"=u32 1888) -> (w374:T4)
        n136 = call "EOL CAN_Send_Single_Message.vi"("Rx Arbitration Id"=u32 1867, "Tx CAN frame"=w374, "Read Session in"=w376, "Write Session in"=w377) -> ("Error out"=w366:errorcluster, "Rx Message"=w368:u8[], "Response Good?"=w369:bool, "TxRx Data"=w370:string[][])  [unwired: 3 in, 1 out]
        n137 = Bundle By Name(cluster=w372, "Event"=w360, "DataBuffer.CAN.TxRx Data"=w370, "DataBuffer.CAN.Response Good?"=w369, "DataBuffer.CAN.Rx Message"=w368, "DataBuffer.error"=w366) -> (w371:T9)
        n138 = call <vilib>:"Add State(s) to Queue__JKI_lib_State_Machine.vi"("State(s) in Front (\"\")"="System: Updata Display" ("State(s) in Front (\"\")"), "State(s) in (\"\")"=w380) -> ("States Out"=w379:string)  [unwired: 13 in]
      }
      frame "Operations: Tester Present" {
        # "Your code here.\n(You can make a copy of, or modify, this frame)"
        n139 = Concatenate Strings(w383, " >> " ("字符串"), w382) -> (w381:string)
        n140 = Unbundle By Name(w393) -> ("DataBuffer.CAN.Write Session in"=w398:refnum<k21>, "DataBuffer.CAN.Read Session in"=w397:refnum<k21>, "DataBuffer.CAN.CAN frame"=w396:T4)
        n141 = Bundle By Name(cluster=w396, "payload"=u8[] [2, 62, 128, 170, 170, 170, 170, 170], "identifier"=u32 1888) -> (w395:T4)
        n142 = call "EOL CAN_Send_Single_Message.vi"("Rx Arbitration Id"=u32 1867, "Tx CAN frame"=w395, "Read Session in"=w397, "Write Session in"=w398) -> ("Error out"=w387:errorcluster, "Rx Message"=w389:u8[], "Response Good?"=w390:bool, "TxRx Data"=w391:string[][])  [unwired: 3 in, 1 out]
        n143 = Bundle By Name(cluster=w393, "Event"=w381, "DataBuffer.CAN.TxRx Data"=w391, "DataBuffer.CAN.Response Good?"=w390, "DataBuffer.CAN.Rx Message"=w389, "DataBuffer.error"=w387) -> (w392:T9)
        n144 = call <vilib>:"Add State(s) to Queue__JKI_lib_State_Machine.vi"("State(s) in Front (\"\")"="System: Updata Display" ("State(s) in Front (\"\")"), "State(s) in (\"\")"=w401) -> ("States Out"=w400:string)  [unwired: 13 in]
      }
      frame "Operations: Request Seed" {
        # "Your code here.\n(You can make a copy of, or modify, this frame)"
        n145 = Concatenate Strings(w404, " >> " ("字符串"), w403) -> (w402:string)
        n146 = Unbundle By Name(w413) -> ("DataBuffer.CAN.Write Session in"=w418:refnum<k21>, "DataBuffer.CAN.Read Session in"=w417:refnum<k21>, "DataBuffer.CAN.CAN frame"=w416:T4)
        n147 = Bundle By Name(cluster=w416, "payload"=u8[] [2, 39, 1, 170, 170, 170, 170, 170]) -> (w415:T4)
        n148 = call "EOL CAN_Send_Single_Message.vi"("Rx Arbitration Id"=u32 1867, "Tx CAN frame"=w415, "Read Session in"=w417, "Write Session in"=w418) -> ("Error out"=w407:errorcluster, "Rx Message"=w409:u8[], "Response Good?"=w410:bool, "TxRx Data"=w411:string[][])  [unwired: 3 in, 1 out]
        n149 = Bundle By Name(cluster=w413, "Event"=w402, "DataBuffer.CAN.TxRx Data"=w411, "DataBuffer.CAN.Response Good?"=w410, "DataBuffer.CAN.Rx Message"=w409, "DataBuffer.error"=w407) -> (w412:T9)
        n150 = call <vilib>:"Add State(s) to Queue__JKI_lib_State_Machine.vi"("State(s) in Front (\"\")"="System: Updata Display" ("State(s) in Front (\"\")"), "State(s) in (\"\")"=w421) -> ("States Out"=w420:string)  [unwired: 13 in]
      }
      frame "Operations: Send Key" {
        # "Your code here.\n(You can make a copy of, or modify, this frame)"
        n151 = Unbundle By Name(w437) -> ("DataBuffer.CAN.Write Session in"=w442:refnum<k21>, "DataBuffer.CAN.Read Session in"=w441:refnum<k21>, "DataBuffer.CAN.CAN frame"=w440:T4, "DataBuffer.CAN.Rx Message"=w427:u8[])
        n152 = Concatenate Strings(w424, " >> " ("字符串"), w423) -> (w422:string)
        n153 = call "Get Key 27 01.vi"("Seed message"=w427) -> ("Key"=w429:u32[])  [unwired: 10 in]
        n154 = Insert Into Array(array=u8[] [6, 39, 2] ("payload"), new element #1=w429, new element #2=u8 170 ("新元素/子数组")) -> (w426:u8[])  [unwired: 1 in]
        n155 = Bundle By Name(cluster=w440, "payload"=w426) -> (w439:T4)
        n156 = call "EOL CAN_Send_Single_Message.vi"("Rx Arbitration Id"=u32 1867, "Tx CAN frame"=w439, "Read Session in"=w441, "Write Session in"=w442) -> ("Error out"=w431:errorcluster, "Rx Message"=w433:u8[], "Response Good?"=w434:bool, "TxRx Data"=w435:string[][])  [unwired: 3 in, 1 out]
        n157 = Bundle By Name(cluster=w437, "Event"=w422, "DataBuffer.CAN.TxRx Data"=w435, "DataBuffer.CAN.Response Good?"=w434, "DataBuffer.CAN.Rx Message"=w433, "DataBuffer.error"=w431) -> (w436:T9)
        n158 = call <vilib>:"Add State(s) to Queue__JKI_lib_State_Machine.vi"("State(s) in Front (\"\")"="System: Updata Display" ("State(s) in Front (\"\")"), "State(s) in (\"\")"=w445) -> ("States Out"=w444:string)  [unwired: 13 in]
      }
      frame "Operations: Check FBL" {
        # "Your code here.\n(You can make a copy of, or modify, this frame)"
        n159 = Concatenate Strings(w448, " >> " ("字符串"), w447) -> (w446:string)
        n160 = Unbundle By Name(w457) -> ("DataBuffer.CAN.Write Session in"=w462:refnum<k21>, "DataBuffer.CAN.Read Session in"=w461:refnum<k21>, "DataBuffer.CAN.CAN frame"=w460:T4)
        n161 = Bundle By Name(cluster=w460, "payload"=u8[] [4, 49, 1, 253, 2, 170, 170, 170]) -> (w459:T4)
        n162 = call "EOL CAN_Send_Single_Message.vi"("Rx Arbitration Id"=u32 1867, "Tx CAN frame"=w459, "Read Session in"=w461, "Write Session in"=w462) -> ("Error out"=w451:errorcluster, "Rx Message"=w453:u8[], "Response Good?"=w454:bool, "TxRx Data"=w455:string[][])  [unwired: 3 in, 1 out]
        n163 = Bundle By Name(cluster=w457, "Event"=w446, "DataBuffer.CAN.TxRx Data"=w455, "DataBuffer.CAN.Response Good?"=w454, "DataBuffer.CAN.Rx Message"=w453, "DataBuffer.error"=w451) -> (w456:T9)
        n164 = call <vilib>:"Add State(s) to Queue__JKI_lib_State_Machine.vi"("State(s) in Front (\"\")"="System: Updata Display" ("State(s) in Front (\"\")"), "State(s) in (\"\")"=w465) -> ("States Out"=w464:string)  [unwired: 13 in]
      }
      frame "Operations: Control DTC" {
        # "Your code here.\n(You can make a copy of, or modify, this frame)"
        n165 = Concatenate Strings(w468, " >> " ("字符串"), w467) -> (w466:string)
        n166 = Unbundle By Name(w478) -> ("DataBuffer.CAN.Write Session in"=w483:refnum<k21>, "DataBuffer.CAN.Read Session in"=w482:refnum<k21>, "DataBuffer.CAN.CAN frame"=w481:T4)
        n167 = Bundle By Name(cluster=w481, "payload"=u8[] [2, 133, 130, 170, 170, 170, 170, 170], "identifier"=u32 1888) -> (w480:T4)
        n168 = call "EOL CAN_Send_Single_Message.vi"("Rx Arbitration Id"=u32 1867, "Tx CAN frame"=w480, "Read Session in"=w482, "Write Session in"=w483) -> ("Error out"=w472:errorcluster, "Rx Message"=w474:u8[], "Response Good?"=w475:bool, "TxRx Data"=w476:string[][])  [unwired: 3 in, 1 out]
        n169 = Bundle By Name(cluster=w478, "Event"=w466, "DataBuffer.CAN.TxRx Data"=w476, "DataBuffer.CAN.Response Good?"=w475, "DataBuffer.CAN.Rx Message"=w474, "DataBuffer.error"=w472) -> (w477:T9)
        n170 = call <vilib>:"Add State(s) to Queue__JKI_lib_State_Machine.vi"("State(s) in Front (\"\")"="System: Updata Display" ("State(s) in Front (\"\")"), "State(s) in (\"\")"=w486) -> ("States Out"=w485:string)  [unwired: 13 in]
      }
      frame "Operations: Comm Control" {
        # "Your code here.\n(You can make a copy of, or modify, this frame)"
        n171 = Concatenate Strings(w491, " >> " ("字符串"), w490) -> (w489:string)
        n172 = Unbundle By Name(w498) -> ("DataBuffer.CAN.Write Session in"=w503:refnum<k21>, "DataBuffer.CAN.Read Session in"=w502:refnum<k21>, "DataBuffer.CAN.CAN frame"=w501:T4)
        n173 = Bundle By Name(cluster=w501, "payload"=u8[] [3, 40, 131, 1, 170, 170, 170, 170]) -> (w500:T4)
        n174 = call "EOL CAN_Send_Single_Message.vi"("Rx Arbitration Id"=u32 1867, "Tx CAN frame"=w500, "Read Session in"=w502, "Write Session in"=w503) -> ("Error out"=w487:errorcluster, "Rx Message"=w494:u8[], "Response Good?"=w495:bool, "TxRx Data"=w496:string[][])  [unwired: 3 in, 1 out]
        n175 = Bundle By Name(cluster=w498, "Event"=w489, "DataBuffer.CAN.TxRx Data"=w496, "DataBuffer.CAN.Response Good?"=w495, "DataBuffer.CAN.Rx Message"=w494, "DataBuffer.error"=w487) -> (w497:T9)
        n176 = call <vilib>:"Add State(s) to Queue__JKI_lib_State_Machine.vi"("State(s) in Front (\"\")"="System: Updata Display" ("State(s) in Front (\"\")"), "State(s) in (\"\")"=w506) -> ("States Out"=w505:string)  [unwired: 13 in]
      }
      frame "Operations: Program Session Request" {
        # "STOP 2.0\nSTRT FD"
        # "Your code here.\n(You can make a copy of, or modify, this frame)"
        n177 = Concatenate Strings(w511, " >> " ("字符串"), w510) -> (w509:string)
        n178 = Unbundle By Name(w519) -> ("DataBuffer.CAN.Write Session in"=w524:refnum<k21>, "DataBuffer.CAN.Read Session in"=w523:refnum<k21>, "DataBuffer.CAN.CAN frame"=w522:T4)
        n179 = Bundle By Name(cluster=w522, "payload"=u8[] [2, 16, 2, 170, 170, 170, 170, 170]) -> (w521:T4)
        n180 = call "EOL CAN_Send_Single_Message.vi"("Msg Wait Time"=u32 1000, "Rx Arbitration Id"=u32 1867, "Tx CAN frame"=w521, "Read Session in"=w523, "Write Session in"=w524) -> ("Error out"=w514:errorcluster, "Rx Message"=w515:u8[], "Response Good?"=w516:bool, "TxRx Data"=w517:string[][])  [unwired: 2 in, 1 out]
        n181 = Bundle By Name(cluster=w519, "Event"=w509, "DataBuffer.CAN.TxRx Data"=w517, "DataBuffer.CAN.Response Good?"=w516, "DataBuffer.CAN.Rx Message"=w515, "DataBuffer.error"=w514) -> (w518:T9)
        n182 = call <vilib>:"Add State(s) to Queue__JKI_lib_State_Machine.vi"("State(s) in Front (\"\")"="System: Updata Display" ("State(s) in Front (\"\")"), "State(s) in (\"\")"=w527) -> ("States Out"=w526:string)  [unwired: 13 in]
      }
      frame "Operations: Program Request Seed" {
        w529 = T5 8 items=["CAN Data"=0, "CAN Remote"=1, "CAN Bus Error"=2, "CAN 2.0 Data"=8, "CAN FD Data"=16, "CAN FD+BRS Data"=24, "J1939 Data"=192, "Delay"=224, "Log Trigger"=225, "Start Trigger"=226] ("type")
        # "Your code here.\n(You can make a copy of, or modify, this frame)"
        n183 = Concatenate Strings(w532, " >> " ("字符串"), w531) -> (w530:string)
        n184 = Unbundle By Name(w541) -> ("DataBuffer.CAN.Write Session in"=w546:refnum<k21>, "DataBuffer.CAN.Read Session in"=w545:refnum<k21>, "DataBuffer.CAN.CAN frame"=w544:T4)
        n185 = Bundle By Name(cluster=w544, "payload"=u8[] [2, 39, 53, 170, 170, 170, 170, 170], "type"=w529) -> (w543:T4)
        n186 = call "EOL CAN_Send_Single_Message.vi"("Msg Wait Time"=u32 1000, "Rx Arbitration Id"=u32 1867, "Tx CAN frame"=w543, "Read Session in"=w545, "Write Session in"=w546) -> ("Error out"=w535:errorcluster, "Rx Message"=w537:u8[], "Response Good?"=w538:bool, "TxRx Data"=w539:string[][])  [unwired: 2 in, 1 out]
        n187 = Bundle By Name(cluster=w541, "Event"=w530, "DataBuffer.CAN.TxRx Data"=w539, "DataBuffer.CAN.Response Good?"=w538, "DataBuffer.CAN.Rx Message"=w537, "DataBuffer.error"=w535) -> (w540:T9)
        n188 = call <vilib>:"Add State(s) to Queue__JKI_lib_State_Machine.vi"("State(s) in Front (\"\")"="System: Updata Display" ("State(s) in Front (\"\")"), "State(s) in (\"\")"=w549) -> ("States Out"=w548:string)  [unwired: 13 in]
      }
      frame "Operations: Program Send Key" {
        w550 = T5 8 items=["CAN Data"=0, "CAN Remote"=1, "CAN Bus Error"=2, "CAN 2.0 Data"=8, "CAN FD Data"=16, "CAN FD+BRS Data"=24, "J1939 Data"=192, "Delay"=224, "Log Trigger"=225, "Start Trigger"=226] ("type")
        # "Your code here.\n(You can make a copy of, or modify, this frame)"
        n189 = Unbundle By Name(w566) -> ("DataBuffer.CAN.Write Session in"=w571:refnum<k21>, "DataBuffer.CAN.Read Session in"=w570:refnum<k21>, "DataBuffer.CAN.CAN frame"=w569:T4, "DataBuffer.CAN.Rx Message"=w556:u8[])
        n190 = Concatenate Strings(w553, " >> " ("字符串"), w552) -> (w551:string)
        n191 = call "Get Key 27 35.vi"("Seed message"=w556) -> ("Key"=w558:u32[])  [unwired: 10 in]
        n192 = Insert Into Array(array=u8[] [6, 39, 54] ("payload"), new element #1=w558, new element #2=u8 170 ("新元素/子数组")) -> (w555:u8[])  [unwired: 1 in]
        n193 = Bundle By Name(cluster=w569, "payload"=w555, "type"=w550) -> (w568:T4)
        n194 = call "EOL CAN_Send_Single_Message.vi"("Rx Arbitration Id"=u32 1867, "Tx CAN frame"=w568, "Read Session in"=w570, "Write Session in"=w571) -> ("Error out"=w560:errorcluster, "Rx Message"=w562:u8[], "Response Good?"=w563:bool, "TxRx Data"=w564:string[][])  [unwired: 3 in, 1 out]
        n195 = Bundle By Name(cluster=w566, "Event"=w551, "DataBuffer.CAN.TxRx Data"=w564, "DataBuffer.CAN.Response Good?"=w563, "DataBuffer.CAN.Rx Message"=w562, "DataBuffer.error"=w560) -> (w565:T9)
        n196 = call <vilib>:"Add State(s) to Queue__JKI_lib_State_Machine.vi"("State(s) in Front (\"\")"="System: Updata Display" ("State(s) in Front (\"\")"), "State(s) in (\"\")"=w574) -> ("States Out"=w573:string)  [unwired: 13 in]
      }
    }
  }
